vi "004 Property node exemple.vi"() -> ()   [LabVIEW 2019]
panel:
  in  "Reset":bool
  in  "Numeric":dbl
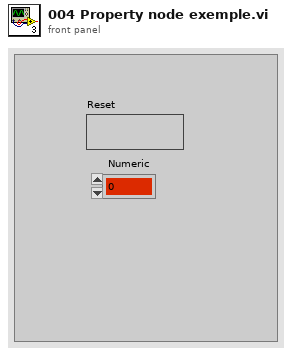
[diagram p1: front panel]
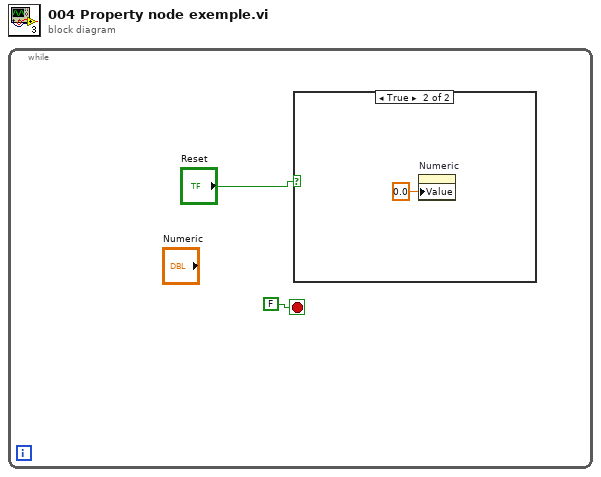
[diagram p0: block diagram]
diagram:
  n1 = while {
    stop <- FALSE stop-if-true
    n2 = case shown="True" "Reset" {
      frame False {
      }
      frame True {
        n3 = property on="Numeric" class="DigNum (strict)"("Value"=0.0 ("Numeric")) -> ()  [unwired: 2 in, 2 out]
      }
    }
  }
